vi "SpinAuxsAuto.vi"(7 "Time":dbl, 8 "error in":errorcluster, 9 "FeedSpd":dbl, 10 "Beltspd":dbl, 11 "ShootSpd":dbl) -> (0 "error out":errorcluster, 3 "Done":bool)   [LabVIEW 2020]
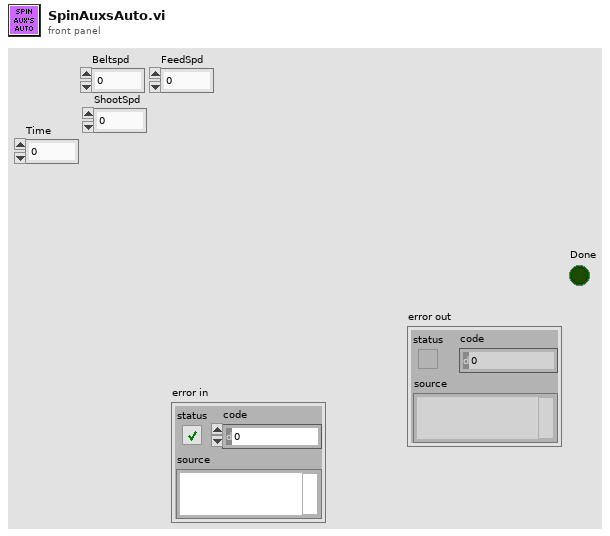
[diagram p1: front panel]
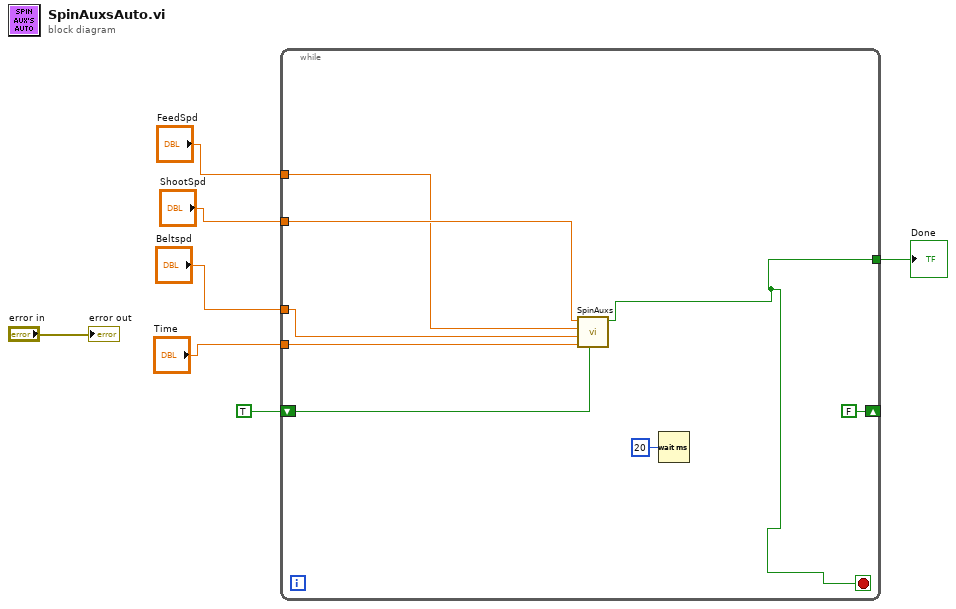
[diagram p0: block diagram]
diagram:
  n1 = while {
    tunnel: [w8] -> w6
    tunnel: "Beltspd" -> [w10]
    tunnel: "ShootSpd" -> [w12]
    tunnel: "FeedSpd" -> [w11]
    shift-right: [FALSE] -> _
    shift-left: TRUE -> [w9]
    tunnel: "Time" -> [w13]
    stop <- w8 stop-if-true
    n2 = call "SpinAuxs.vi"("Init"=w9, "Time"=w13, "BeltSpeed"=w10, "FeederSpeed"=w11, "ShootSpeed"=w12) -> ("Finished"=w8:bool)  [unwired: 5 in, 1 out]
    n3 = Wait (ms)(milliseconds to wait=u32 20) -> ()  [unwired: 1 out]
  }
  "Done" <- w6
  "error out" <- "error in"
